vi "Log The Message.vi"(11 "Square Message":refnum<class "Square Message.lvclass">) -> (2 "log text":string="Draw Square")   [LabVIEW 2019, in "Draw Messages.lvlib" / "Square Message.lvclass"]
uses:
  Square Message.lvclass
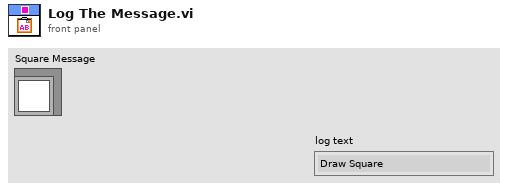
[diagram p1: front panel]
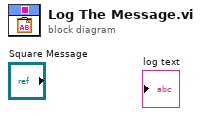
[diagram p0: block diagram]
diagram:
